vi "Replace LocalHost with IP.vi"(8 "error in (no error)":errorcluster, 10 "IP Address":string, 11 "URL":string) -> (0 "error out":errorcluster, 3 "URL with IP":string)   [LabVIEW 2017, in "Shared Variables CD 2.0 Configuration.lvlib"]
uses:
  Shared Variables CD 2.0 Configuration.lvlib
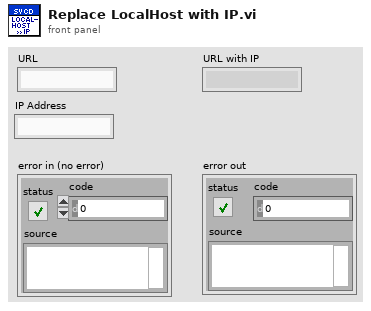
[diagram p1: front panel]
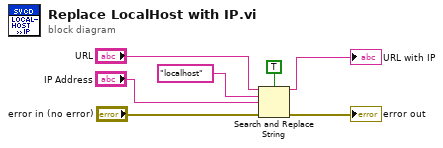
[diagram p0: block diagram]
diagram:
  n1 = Search and Replace String(case sensitive?=TRUE ("ignore case? (F)"), input string="URL", search string="localhost", replace string="IP Address", error in="error in (no error)") -> (result string=→"URL with IP":string, error out=→"error out":errorcluster)  [unwired: 3 in, 2 out]
